vi "adjust.vi"(8 "error in (no error)":errorcluster, 11 "LightSourceMH110124MaiTai in":refnum<class "LightSourceMH110124MaiTai.lvclass">) -> (0 "error out":errorcluster, 3 "LightSourceMH110124MaiTai out":refnum<class "LightSourceMH110124MaiTai.lvclass">)   [LabVIEW 2010, in "LightSourceMH110124MaiTai.lvclass"]
uses:
  LightSourceMH110124MaiTai.lvclass
  LightSourceMH110124MaiTai.lvclass/LightSourceMH110124MaiTai.ctl
  class_data.vi
  common/classes/ErrorController/ErrorController/class_data.vi
  common/classes/ErrorController/ErrorController/ErrorController.lvclass
panel:
  out "humidity":dbl caption="%"
  in  "initialise?":bool
  in  "switch off":bool
  in  "shutter":bool
  out "pulsing":bool
  in  "stop":bool
  out "get wavelength":dbl[unit](slide)
  out "power":dbl[unit](slide) scale=0.0..4.0
  in  "wavelength":i32(slide) scale=690.0..1040.0
  in  "safe mode":bool
  # "laser"
  # "humidity"
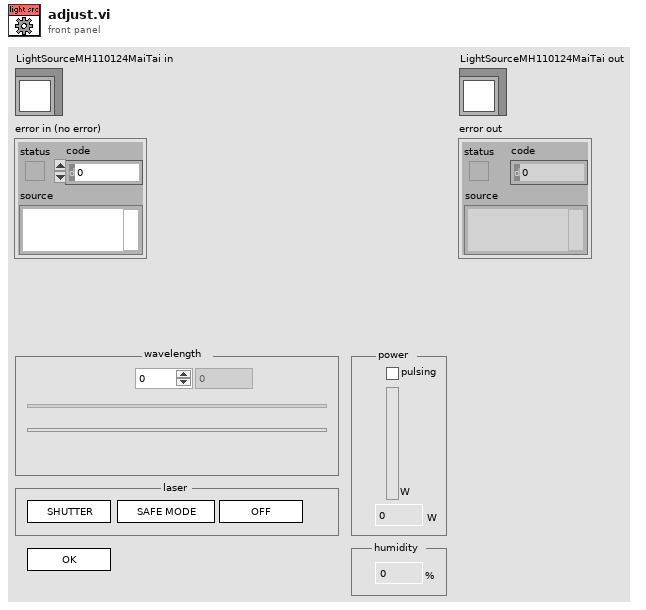
[diagram p1: front panel]
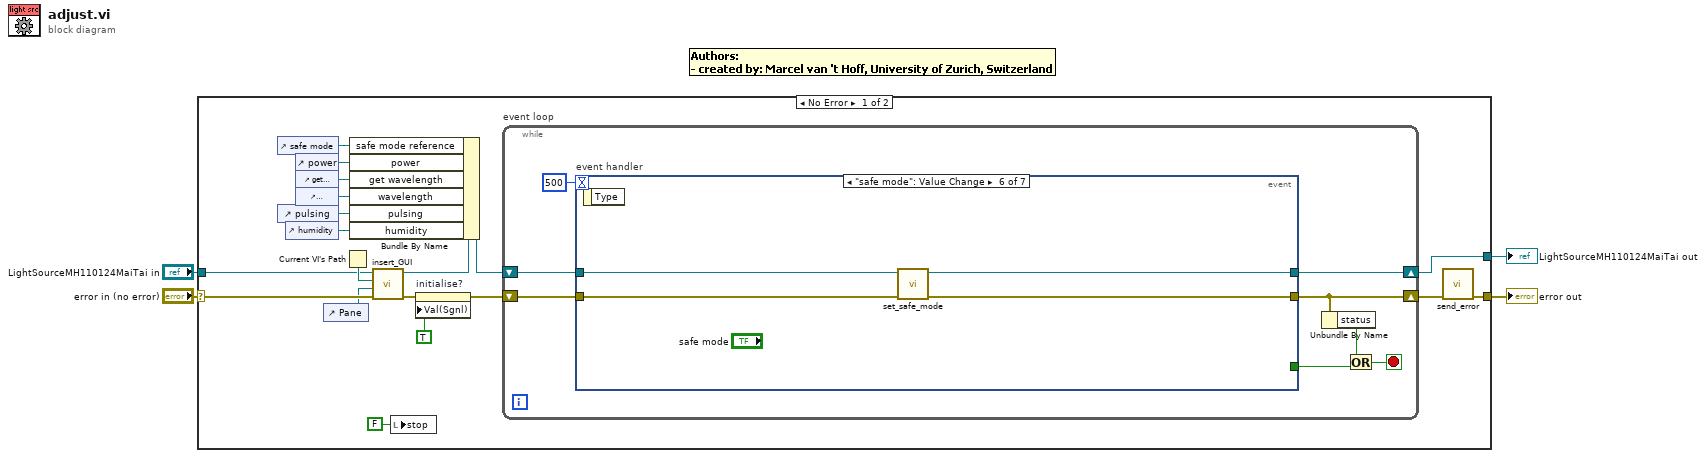
[diagram p0: block diagram]
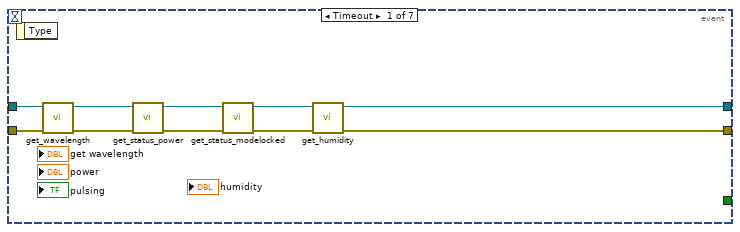
[diagram p2: hidden frame]
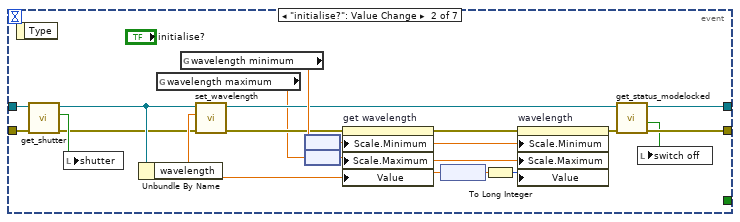
[diagram p3: hidden frame]
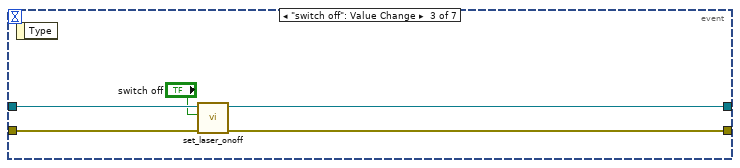
[diagram p4: hidden frame]
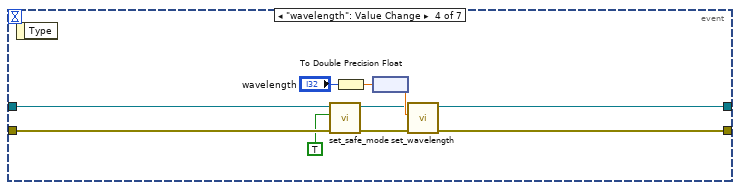
[diagram p5: hidden frame]
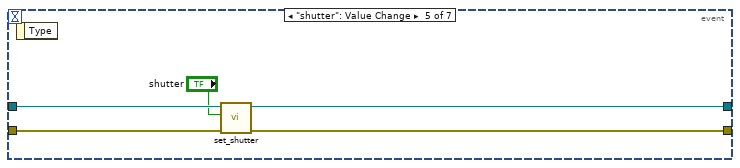
[diagram p6: hidden frame]
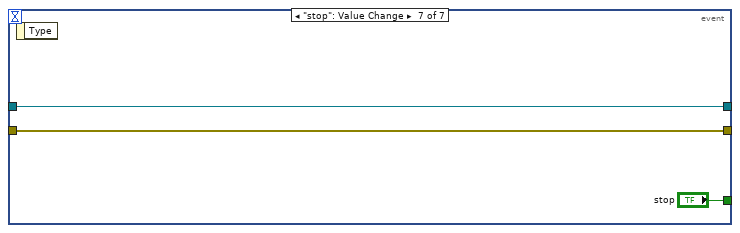
[diagram p7: hidden frame]
diagram:
  n1 = case shown="No Error" "error in (no error)" {
    selector: "error in (no error)" -> [w20 w89]
    tunnel: [w13 w89] -> w3
    tunnel: [w23 w88] -> w2
    tunnel: "LightSourceMH110124MaiTai in" -> [w21 w88]
    frame No Error {
      n2 = control-ref of="safe mode"() -> (w10:refnum<vi>)
      n3 = control-ref of="pulsing"() -> (w6:refnum<vi>)
      n4 = control-ref of="humidity"() -> (w5:refnum<vi>)
      n5 = control-ref of="power"() -> (w9:refnum<vi>)
      n6 = control-ref of="get wavelength"() -> (w7:refnum<vi>)
      n7 = control-ref of="wavelength"() -> (w8:refnum<vi>)
      n8 = control-ref of="Pane"() -> (w19:refnum<vi>)
      n9 = Current VI's Path() -> (path=w22:path)
      n10 = call-dynamic "insert_GUI.vi"("error in (no error)"=w20, "Pane"=w19, "VI path"=w22, "GenericComponent in"=w21) -> ("error out"=w17:errorcluster, "GenericComponent out"=w12:refnum<class "LightSourceMH110124MaiTai.lvclass">)  [unwired: 6 in]
      n11 = Bundle By Name(cluster=w12, "safe mode reference"=w10, "power"=w9, "get wavelength"=w7, "wavelength"=w8, "pulsing"=w6, "humidity"=w5) -> (w11:refnum<class "LightSourceMH110124MaiTai.lvclass">)
      n12 = local write "stop"(FALSE ("stop")) -> ()
      n13 = property on="initialise?" class="Bool (strict)"(error in=w17, "Val(Sgnl)"=TRUE ("stop")) -> (error out=w16:errorcluster)  [unwired: 1 in, 1 out]
      n14 = while "event loop" {
        shift-right: [w28] -> w14
        shift-left: w16 -> [w29]
        shift-right: [w31] -> w23
        shift-left: w11 -> [w30]
        stop <- w26 stop-if-true
        n15 = event "event handler" shown="[5] \"safe mode\": Value Change" {
          selector: _ -> [_ _ _ _ _ _ _]
          dyn-events: _ -> [_ _ _ _ _ _ _]
          timeout: 500 -> [_ _ _ _ _ _ _]
          tunnel: [w34 w54 w64 w71 w77 w83 w87] -> w31
          tunnel: w30 -> [w41 w59 w65 w70 w80 w84 w87]
          tunnel: [w32 w52 w63 w72 w76 w81 w86] -> w28
          tunnel: w29 -> [w40 w58 w62 w68 w79 w82 w86]
          tunnel: [_ _ _ _ _ _ "stop"] -> w25
          event Timeout {
            n16 = event-data() -> ()  [unwired: 1 in, 1 out]
            n17 = call-dynamic "get_wavelength.vi"("error in (no error)"=w40, "LightSourceMH110124MaiTai in"=w41) -> ("error out"=w39:errorcluster, "LightSourceMH110124MaiTai out"=w38:refnum<class "LightSourceMH110124MaiTai.lvclass">)  [unwired: 7 in, 1 out]
            n18 = call-dynamic "get_status_power.vi"("error in (no error)"=w39, "LightSourceMH110124MaiTai in"=w38) -> ("error out"=w36:errorcluster, "LightSourceMH110124MaiTai out"=w37:refnum<class "LightSourceMH110124MaiTai.lvclass">)  [unwired: 7 in, 1 out]
            n19 = call-dynamic "get_status_modelocked.vi"("error in (no error)"=w36, "LightSourceMH110124MaiTai in"=w37) -> ("error out"=w33:errorcluster, "LightSourceMH110124MaiTai out"=w35:refnum<class "LightSourceMH110124MaiTai.lvclass">)  [unwired: 6 in, 2 out]
            n20 = call-dynamic "get_humidity.vi"("error in (no error)"=w33, "LightSourceMH110124MaiTai in"=w35) -> ("error out"=w32:errorcluster, "LightSourceMH110124MaiTai out"=w34:refnum<class "LightSourceMH110124MaiTai.lvclass">)  [unwired: 7 in, 1 out]
          }
          event "initialise?": Value Change {
            n21 = event-data() -> ()  [unwired: 1 in, 1 out]
            n22 = call-dynamic "get_shutter.vi"("error in (no error)"=w58, "LightSourceMH110124MaiTai in"=w59) -> ("error out"=w42:errorcluster, "shutter open out?"=w60:bool, "LightSourceMH110124MaiTai out"=w43:refnum<class "LightSourceMH110124MaiTai.lvclass">)  [unwired: 7 in]
            n23 = local write "shutter"(w60) -> ()
            n24 = Unbundle By Name(w43) -> ("wavelength"=w48:dbl[unit])
            n25 = global read "class_data.vi" "wavelength maximum"() -> (w44:dbl[unit])
            n26 = global read "class_data.vi" "wavelength minimum"() -> (w47:dbl[unit])
            n27 = call-dynamic "set_wavelength.vi"("error in (no error)"=w42, "wavelength in"=w48, "LightSourceMH110124MaiTai in"=w43) -> ("error out"=w46:errorcluster, "LightSourceMH110124MaiTai out"=w45:refnum<class "LightSourceMH110124MaiTai.lvclass">)  [unwired: 7 in]
            n28 = node(w47) -> (w57:dbl)
            n29 = node(w44) -> (w56:dbl)
            n30 = property on="get wavelength" class="Slide (strict)"(error in=w46, "Scale.Minimum"=w57, "Scale.Maximum"=w56, "Value"=w48) -> (error out=w55:errorcluster)  [unwired: 1 in, 1 out]
            n31 = node(w48) -> (w50:dbl)
            n32 = To Long Integer(number=w50) -> (32bit integer=w51:i32)
            n33 = property on="wavelength" class="Slide (strict)"(error in=w55, "Scale.Minimum"=w57, "Scale.Maximum"=w56, "Value"=w51) -> (error out=w53:errorcluster)  [unwired: 1 in, 1 out]
            n34 = call-dynamic "get_status_modelocked.vi"("error in (no error)"=w53, "LightSourceMH110124MaiTai in"=w45) -> ("error out"=w52:errorcluster, "Emission"=w49:bool, "LightSourceMH110124MaiTai out"=w54:refnum<class "LightSourceMH110124MaiTai.lvclass">)  [unwired: 6 in, 1 out]
            n35 = local write "switch off"(w49) -> ()
          }
          event "switch off": Value Change {
            n36 = event-data() -> ()  [unwired: 1 in, 1 out]
            n37 = call-dynamic "set_laser_onoff.vi"("error in (no error)"=w62, "on?"="switch off", "LightSourceMH110124MaiTai in"=w65) -> ("error out"=w63:errorcluster, "LightSourceMH110124MaiTai out"=w64:refnum<class "LightSourceMH110124MaiTai.lvclass">)  [unwired: 7 in]
          }
          event "wavelength": Value Change {
            n38 = event-data() -> ()  [unwired: 1 in, 1 out]
            n39 = call-dynamic "set_safe_mode.vi"("error in (no error)"=w68, "exit safe mode? (F)"=TRUE ("exit safe mode?"), "LightSourceMH110124MaiTai in"=w70) -> ("error out"=w67:errorcluster, "LightSourceMH110124MaiTai out"=w69:refnum<class "LightSourceMH110124MaiTai.lvclass">)  [unwired: 7 in]
            n40 = To Double Precision Float(number="wavelength") -> (double precision float=w73:dbl)
            n41 = node(w73) -> (w74:dbl[unit])
            n42 = call-dynamic "set_wavelength.vi"("error in (no error)"=w67, "wavelength in"=w74, "LightSourceMH110124MaiTai in"=w69) -> ("error out"=w72:errorcluster, "LightSourceMH110124MaiTai out"=w71:refnum<class "LightSourceMH110124MaiTai.lvclass">)  [unwired: 7 in]
          }
          event "shutter": Value Change {
            n43 = event-data() -> ()  [unwired: 1 in, 1 out]
            n44 = call-dynamic "set_shutter.vi"("error in (no error)"=w79, "shutter open?"="shutter", "LightSourceMH110124MaiTai in"=w80) -> ("error out"=w76:errorcluster, "LightSourceMH110124MaiTai out"=w77:refnum<class "LightSourceMH110124MaiTai.lvclass">)  [unwired: 6 in, 1 out]
          }
          event "safe mode": Value Change {
            n45 = event-data() -> ()  [unwired: 1 in, 1 out]
            n46 = call-dynamic "set_safe_mode.vi"("error in (no error)"=w82, "LightSourceMH110124MaiTai in"=w84) -> ("error out"=w81:errorcluster, "LightSourceMH110124MaiTai out"=w83:refnum<class "LightSourceMH110124MaiTai.lvclass">)  [unwired: 8 in]
          }
          event "stop": Value Change {
            n47 = event-data() -> ()  [unwired: 1 in, 1 out]
          }
        }
        n48 = Unbundle By Name(w28) -> ("status"=w27:bool)
        n49 = Or(x=w27, y=w25) -> (x .or. y?=w26:bool)
      }
      n50 = call "send_error.vi"("error in (no error)"=w14) -> ("error out"=w13:errorcluster)  [unwired: 10 in]
    }
    frame Error {
    }
  }
  "error out" <- w3
  "LightSourceMH110124MaiTai out" <- w2
